vi "Read Instrument.vi"(8 "error in (no error)":errorcluster, 11 "Instrument UI in":refnum<class "Instrument UI.lvclass">) -> (0 "error out":errorcluster, 2 "Instrument":refnum<class "Instrument.lvclass">, 3 "Instrument UI":refnum<class "Instrument UI.lvclass">)   [LabVIEW 2019, in "Instrument.lvlib" / "Instrument UI.lvclass"]
uses:
  Instrument UI.lvclass
  Instrument/Instrument.lvclass
  Instrument UI.lvclass/Instrument UI.ctl
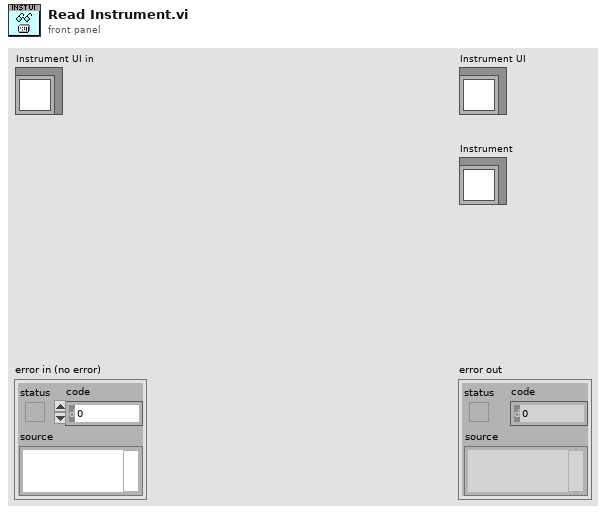
[diagram p1: front panel]
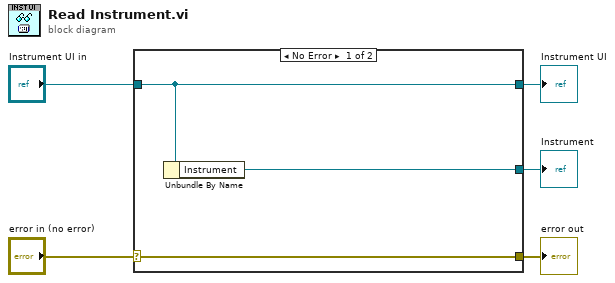
[diagram p0: block diagram]
diagram:
  n1 = case shown="No Error" "error in (no error)" {
    selector: "error in (no error)" -> [w8 w9]
    tunnel: [w8 w9] -> w4
    tunnel: [w7 w10] -> w2
    tunnel: "Instrument UI in" -> [w7 w10]
    tunnel: [w6 _] -> w1
    frame No Error {
      n2 = Unbundle By Name(w7) -> ("Instrument"=w6:refnum<class "Instrument.lvclass">)
    }
    frame Error {
    }
  }
  "error out" <- w4
  "Instrument UI" <- w2
  "Instrument" <- w1
